vi "Waveform Convert 4C.vi"(7 "BlockID":u32, 8 "error in":errorcluster, 11 "Waveform Array":sgl[][](array[numeric])) -> (0 "error out":errorcluster, 1 "ModWfms":string)   [LabVIEW 2012, in "Data Acquisition.lvlib" / "DAQ Actor.lvclass"]
uses:
  DAQ Actor.lvclass
  Common/Controls/Modified Waveform.ctl
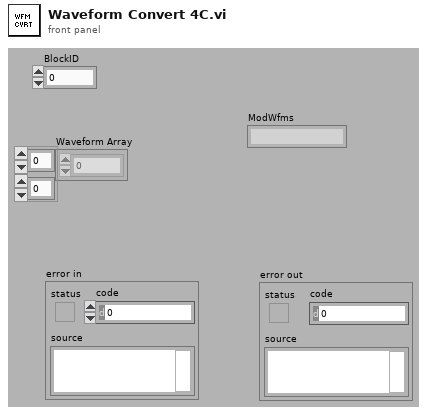
[diagram p1: front panel]
types:
  T1 = enum16{"big-endian, network order", "native, host order", "little-endian"}
  T2 = typedef "Modified Waveform.ctl" = cluster{"BlockID":u32, "to (s)":dbl, "Y":sgl[][]}
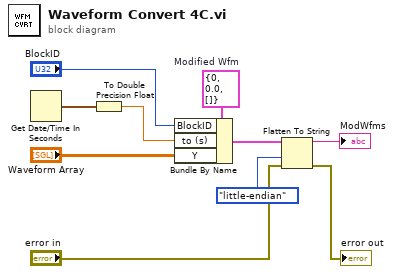
[diagram p0: block diagram]
diagram:
  w10 = T2 {"BlockID"=0, "to (s)"=0.0, "Y"=[]}  # Modified Wfm
  n1 = Get Date/Time In Seconds() -> (seconds since 1Jan1904=w4:timestamp)
  n2 = To Double Precision Float(number=w4) -> (double precision float=w3:dbl)
  n3 = Bundle By Name(cluster=w10, "BlockID"="BlockID", "to (s)"=w3, "Y"="Waveform Array") -> (w9:T2)
  n4 = Flatten To String(anything=w9, byte order (0:big-endian, network order)=T1."little-endian", error in (no error)="error in") -> (data string=→"ModWfms":string, error out=→"error out":errorcluster)  [unwired: 1 in, 1 out]
